vi "Image Stitching.vi"() -> ()   [LabVIEW 2017]
uses:
  <vilib>/vision/NI_Vision_Development_Module.lvlib
panel:
  out "Stiched Image":T1(plugin-control)
  out "Image 2":T1(plugin-control)
  out "Image 1":T1(plugin-control)
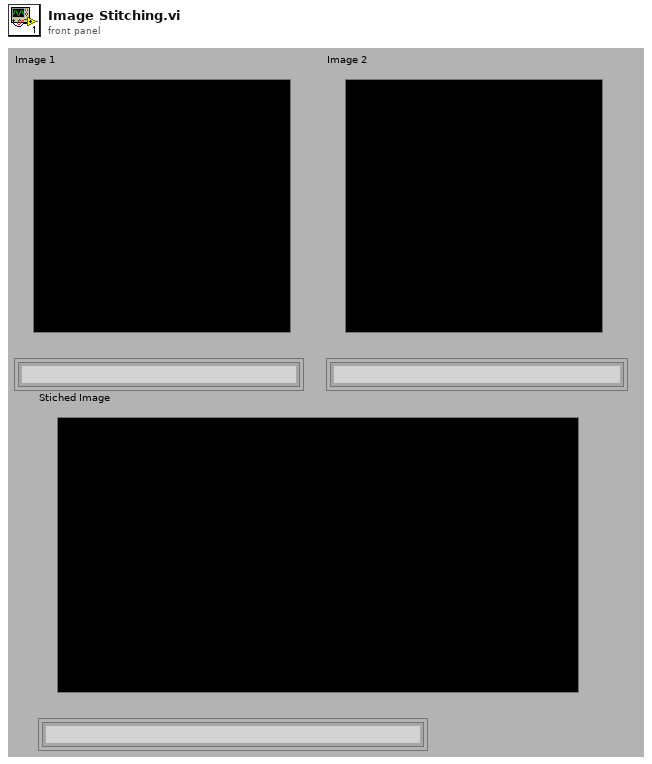
[diagram p1: front panel]
types:
  T1 = typedef "IMAQ Image.ctl" = refnum<image>
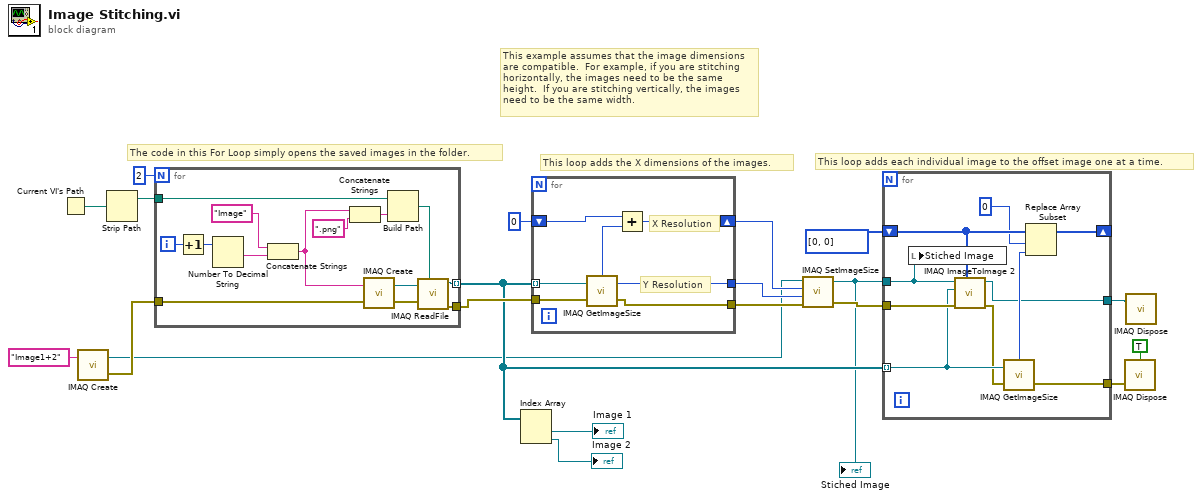
[diagram p0: block diagram]
diagram:
  # "This loop adds each individual image to the offset image one at a time."
  # "This loop adds the X dimensions of the images."
  # "This example assumes that the image dimensions\nare compatible.  For example, if you are stitching\nhorizontally, the images need to be the same\nheight.  If you are stitching vertically, the images\nneed to be the same width."
  # "The code in this For Loop simply opens the saved images in the folder."
  n1 = Current VI's Path() -> (path=w19:path)
  n2 = call "IMAQ Create"("Image Name"="Image1+2") -> ("New Image"=w2:T1, "error out"=w17:errorcluster)  [unwired: 3 in, 1 out]
  n3 = Strip Path(path=w19) -> (stripped path=w18:path)  [unwired: 1 out]
  n4 = for {
    N: 2 -> [_]
    tunnel: w18 -> [w32]
    tunnel: [w26] -> w8 mode=indexing
    tunnel: [w25] -> w14
    tunnel: w17 -> [w24]
    i -> [w31]
    n5 = Increment(x=w31) -> (x+1=w30:i32)
    n6 = Number To Decimal String(number=w30) -> (decimal integer string=w34:string)  [unwired: 1 out]
    n7 = Concatenate Strings("Image", w34) -> (w21:string)
    n8 = Concatenate Strings(w21, ".png") -> (w23:string)
    n9 = call "IMAQ Create"("Image Name"=w21, "error in (no error)"=w24) -> ("New Image"=w28:T1, "error out"=w29:errorcluster)  [unwired: 2 in, 1 out]
    n10 = Build Path(base path=w32, name or relative path=w23) -> (appended path=w27:path)
    n11 = call "IMAQ ReadFile"("File Path"=w27, "error in (no error)"=w29, "Image"=w28) -> ("error out"=w25:errorcluster, "Image Out"=w26:T1)  [unwired: 2 in, 5 out]
  }
  n12 = Index Array(array=w8) -> (element #1=→"Image 1":T1, element #2=→"Image 2":T1)  [unwired: 2 in]
  n13 = for {
    tunnel: w8 -> [w41] mode=indexing
    shift-right: [w39] -> w12
    shift-left: 0 ("Y Resolution") -> [w40]
    tunnel: w14 -> [w38]
    tunnel: [w37] -> w11
    tunnel: [w36] -> w13
    # "Y Resolution"
    # "X Resolution"
    n14 = call "IMAQ GetImageSize"("Image"=w41, "error in (no error)"=w38) -> ("Y Resolution"=w37:i32, "X Resolution"=w35:i32, "error out"=w36:errorcluster)  [unwired: 2 out]
    n15 = Add(x=w40, y=w35) -> (x+y=w39:i32)
  }
  n16 = call "IMAQ SetImageSize"("error in (no error)"=w13, "Y Resolution"=w11, "X Resolution"=w12, "Image"=w2) -> ("error out"=w10:errorcluster, "Image Out"=w1:T1)  [unwired: 1 out]
  "Stiched Image" <- w1
  n17 = for {
    tunnel: w8 -> [w50] mode=indexing
    tunnel: w1 -> [w42]
    tunnel: w10 -> [w51]
    tunnel: [w43] -> w3
    shift-right: [w48] -> _
    shift-left: i32[] [0, 0] -> [w47]
    tunnel: [w44] -> w5
    n18 = local write "Stiched Image"(w42) -> ()
    n19 = call "IMAQ ImageToImage 2"("Offset Left/Top"=w47, "error in (no error)"=w51, "Image Src (Small)"=w50, "Image Src (Large)"=w42) -> ("error out"=w45:errorcluster, "Image Dst Out"=w43:T1)  [unwired: 2 in, 4 out]
    n20 = call "IMAQ GetImageSize"("Image"=w50, "error in (no error)"=w45) -> ("X Resolution"=w49:i32, "error out"=w44:errorcluster)  [unwired: 3 out]
    n21 = Replace Array Subset(array=w47, new element=w49, index=0) -> (w48:i32[])
  }
  n22 = call "IMAQ Dispose"("All Images? (No)"=TRUE, "error in (no error)"=w5) -> ()  [unwired: 1 in, 4 out]
  n23 = call "IMAQ Dispose"("Image"=w3) -> ()  [unwired: 5 in, 1 out]
